vi "ctrlHeadingOnWP.vi"(1 "p(t)":dbl[](array[numeric]), 3 "psi":dbl, 4 "pathCoords":cluster{"x":dbl, "y":dbl}[](array[cluster]), 8 "u":dbl[](array[numeric])) -> (10 "45degrees":bool, 11 "e_psi":dbl, 12 "psiplot":cluster{"psi_d":dbl, "psi":dbl}, 13 "e":dbl, 15 "eta_i 2":dbl[](array[numeric]), 16 "WithinProximity radius":bool, 17 "eta_r":dbl[](array[numeric]), 19 "delta":dbl, 20 "iOut":dbl, 23 "U":dbl[](array[numeric]))   [LabVIEW 2014]
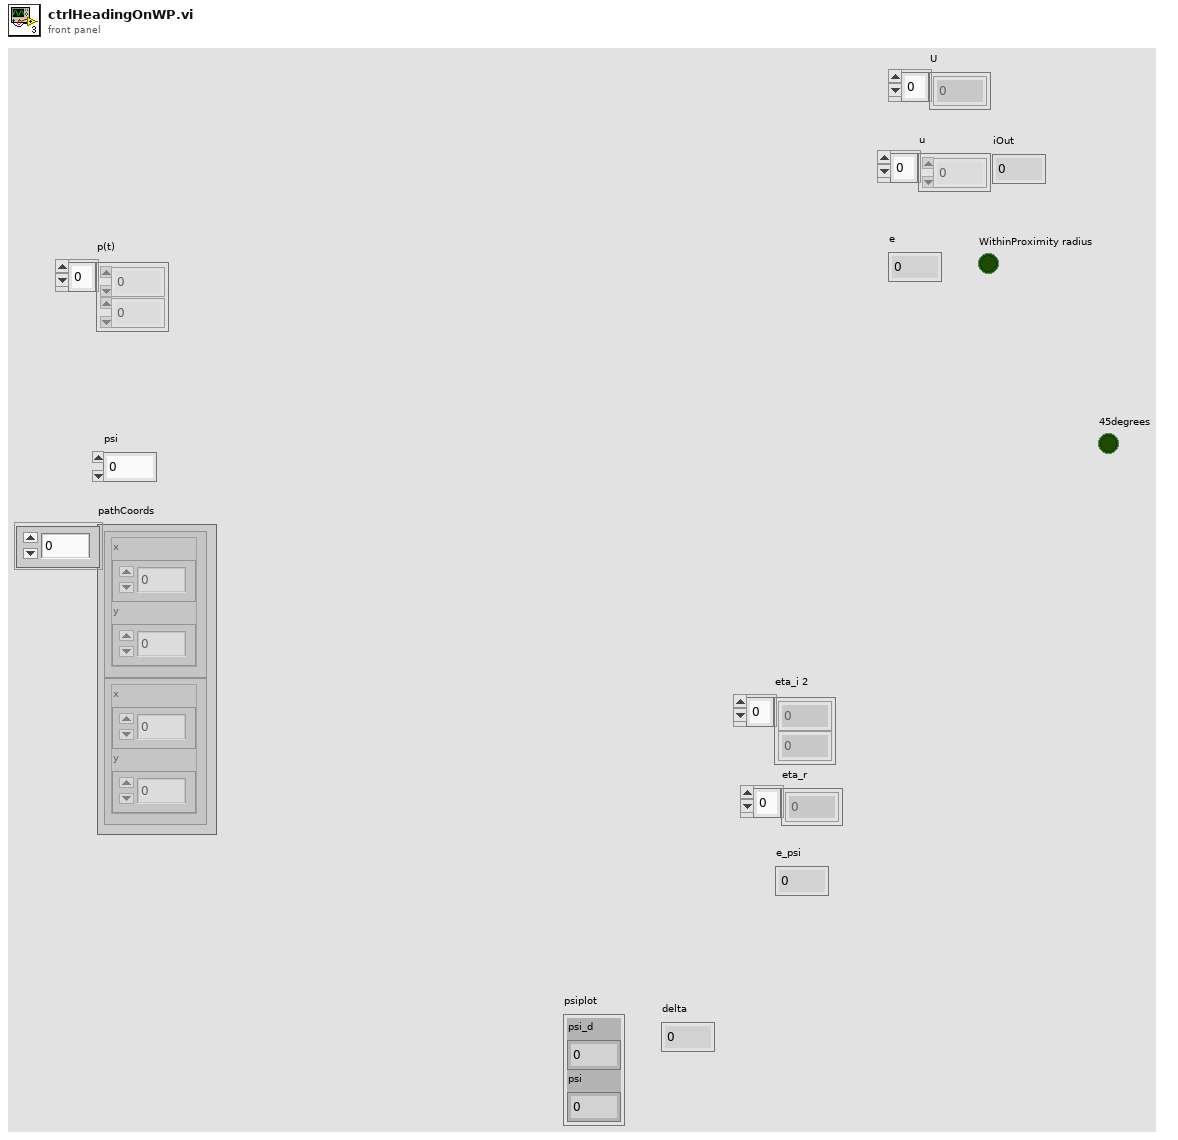
[diagram p1: front panel]
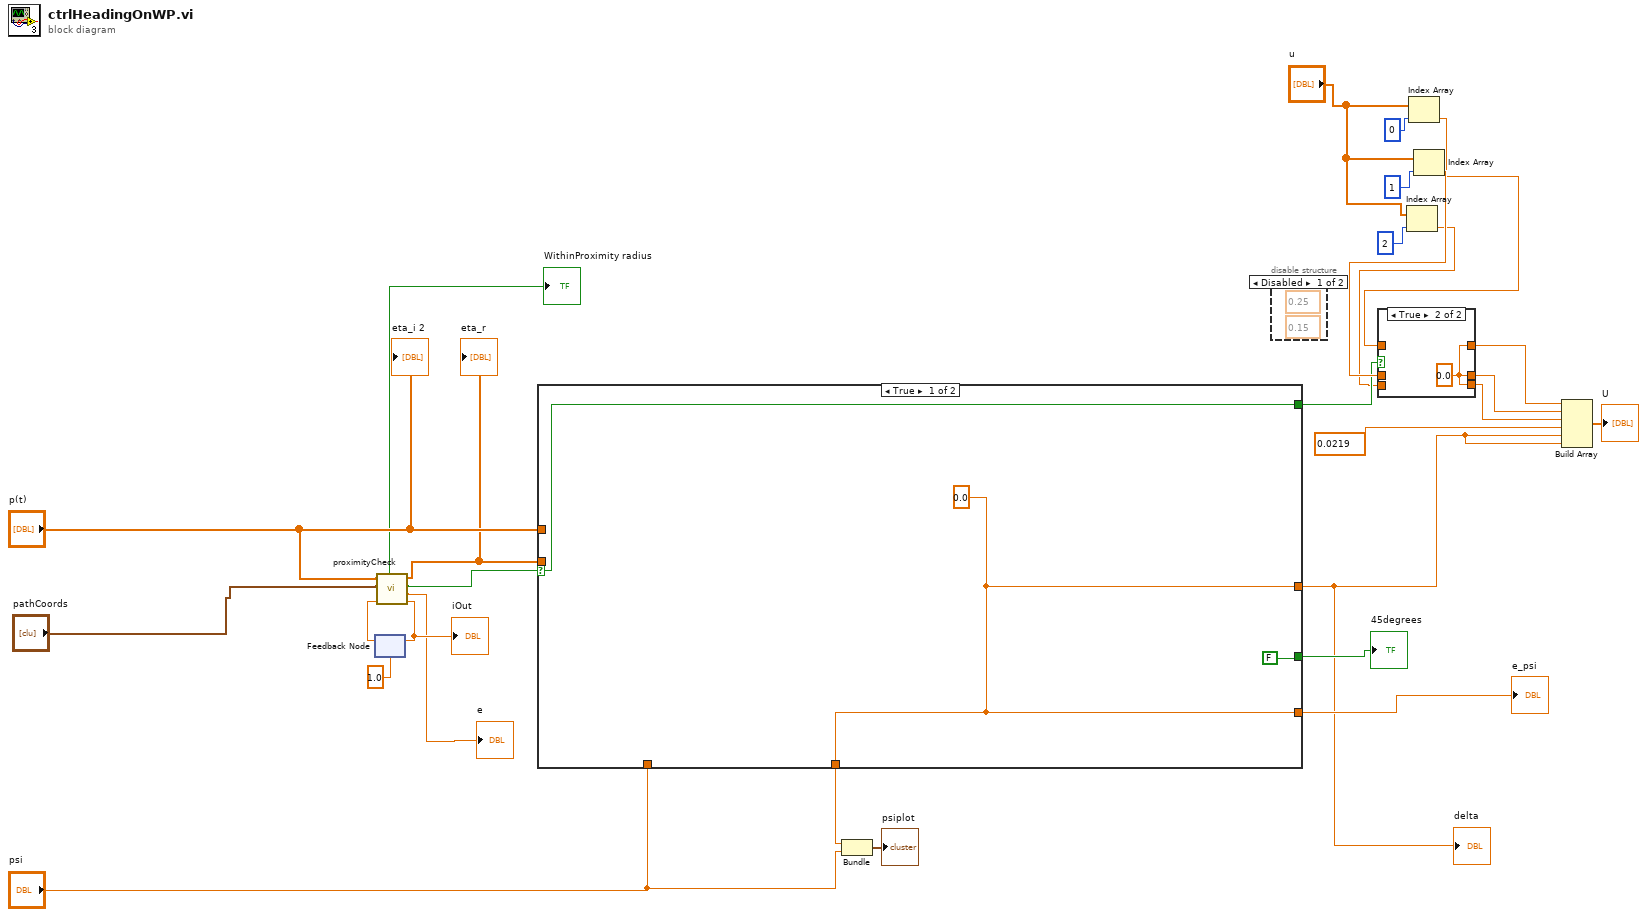
[diagram p0: block diagram]
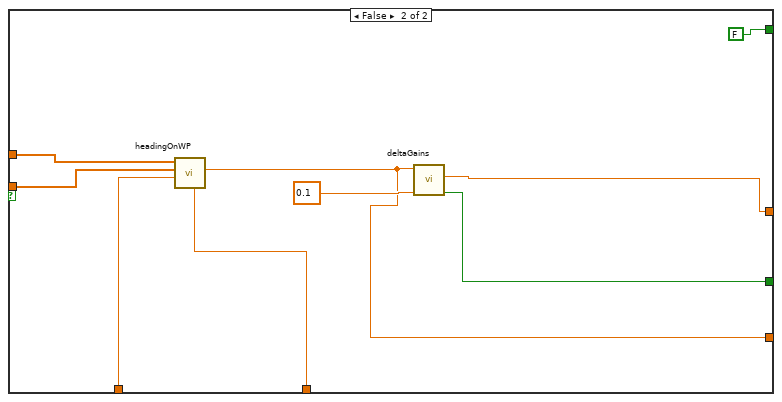
[diagram p4: hidden frame]
diagram:
  n1 = feedback #1(1.0 ("iOut")) -> (w23:dbl)
  n2 = call "proximityCheck.vi"("i"=w23, "pathCoords"="pathCoords", "p(t)"="p(t)") -> ("iOut"=w24:dbl, "e"=→"e":dbl, "indexOutOfBounds"=w19:bool, "p_d"=w20:dbl[], "WithinProximity radius"=→"WithinProximity radius":bool)  [unwired: 1 in]
  "eta_r" <- w20
  "iOut" <- w24
  n3 = feedback-in #1(w24) -> ()
  n4 = case shown="True" w19 {
    selector: w19 -> [w30 _]
    tunnel: "psi" -> [_ w35]
    tunnel: "p(t)" -> [_ w40]
    tunnel: [w31 w33] -> w1
    tunnel: w20 -> [_ w39]
    tunnel: [w31 w34] -> w27
    tunnel: [w31 w32] -> w15
    tunnel: [w30 FALSE] -> w7
    tunnel: [FALSE w36] -> w6
    frame True {
      w31 = 0.0
    }
    frame False {
      n5 = call "headingOnWP.vi"("psi"=w35, "p_d"=w39, "pt"=w40) -> ("e_psi"=w34:dbl, "psi_d"=w32:dbl)  [unwired: 7 in]
      n6 = call "deltaGains.vi"("Kp"=0.1 ("iOut"), "e_psi"=w34) -> ("45degrees"=w36:bool, "delta"=w33:dbl)  [unwired: 8 in]
    }
  }
  "e_psi" <- w27
  "45degrees" <- w6
  "delta" <- w1
  n7 = Bundle("psi_d"=w15, "psi"="psi") -> (→"psiplot":cluster{"psi_d":dbl, "psi":dbl})  [unwired: 1 in]
  n8 = disable-structure shown="Disabled" {
    frame Disabled {
      (unwired) 0.15
      (unwired) 0.25
    }
    frame Enabled {
    }
  }
  n9 = Index Array(array="u", index=2) -> (element=w4:dbl)
  n10 = Index Array(array="u", index=0) -> (element=w8:dbl)
  n11 = Index Array(array="u", index=1) -> (element=w9:dbl)
  n12 = case shown="True" w7 {
    tunnel: [w43 w44] -> w11
    tunnel: [w42 w44] -> w10
    tunnel: w9 -> [w43 _]
    tunnel: w8 -> [w42 _]
    tunnel: [w41 w44] -> w3
    tunnel: w4 -> [w41 _]
    frame False {
    }
    frame True {
      w44 = 0.0
    }
  }
  n13 = Build Array(w10, w11, w3, 0.0219, w1, w1) -> (→"U":dbl[])
  "eta_i 2" <- "p(t)"
